vi "Day1-b.vi"(10 "Input":string="15931\n8782\n16940\n14614\n\n4829\n12415\n13259\n11441\n8199\n\n2540\n2500\n6341\n2235\n1858\n4157\n5053\n6611\n1050\n4401\n6187\n1078\n3297\n\n25264\n23014\n15952\n\n10156\n4544\n4930\n11786\n15822\n\n1264\n6399\n2031\n6892\n3115\n5151\n5093\n6724\n7001\n4011\n1458\n1945\n\n2106\n2016\n1528\n2524\n6089\n4466\n3154\n2686\n3289\n5831\n1520\n2122\n5744\n\n33066\n22616\n\n1993\n8485\n1037\n9730\n2076\n7492\n10000\n2971\n\n11027\n9137\n4599\n7461\n1531\n12939\n\n17530\n18837\n19466\n4845\n\n1467\n4870\n10176\n6657\n5608\n2096\n9977\n6478\n\n18828\n26577\n\n17901\n5059\n13789\n4993\n\n6676\n3415\n2464\n5937\n4275\n6629\n7566\n1943\n6313\n4572\n\n9121\n10713\n5071\n1669\n7736\n10522\n6231\n\n6400\n1771\n4568\n7681\n7486\n60...") -> (2 "Output":i32)   [LabVIEW 2017]
uses:
  OOP/Elf/Elf.lvclass
  OOP/ElfHeap/ElfHeap.lvclass
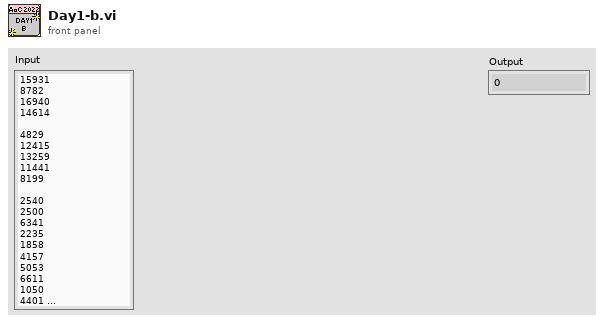
[diagram p1: front panel]
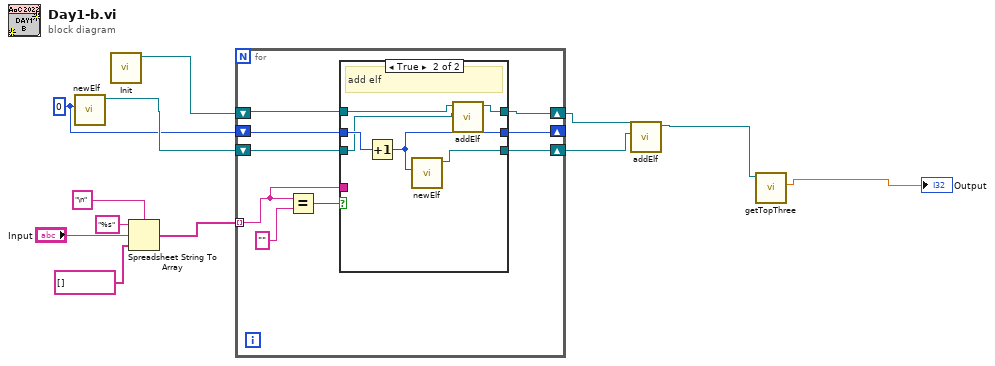
[diagram p0: block diagram]
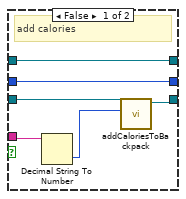
[diagram p2: hidden frame]
diagram:
  w6 = 0 ("Index")
  n1 = call "newElf.vi"("Index"=w6) -> ("Elf out"=w7:refnum<class "Elf.lvclass">)  [unwired: 9 in, 1 out]
  n2 = call "Init.vi"() -> ("ElfHeap out"=w5:refnum<class "ElfHeap.lvclass">)  [unwired: 10 in, 1 out]
  n3 = Spreadsheet String To Array(delimiter (Tab)="\n", format string="%s", spreadsheet string="Input", array type (2D Dbl)=string[] []) -> (array=w9:string[])
  n4 = for {
    tunnel: w9 -> [w13] mode=indexing
    shift-right: [w19] -> w4
    shift-left: w5 -> [w18]
    shift-right: [w16] -> _
    shift-left: w6 -> [w15]
    shift-right: [w14] -> w3
    shift-left: w7 -> [w17]
    n5 = Equal?(x=w13, y="" ("delimiter (Tab)")) -> (x = y?=w20:bool)
    n6 = case shown="True" w20 {
      tunnel: [w27 w28] -> w19
      tunnel: w18 -> [w27 w30]
      tunnel: w17 -> [w25 w29]
      tunnel: [w26 w32] -> w16
      tunnel: w15 -> [w26 w33]
      tunnel: [w24 w31] -> w14
      tunnel: w13 -> [w23 _]
      frame False {
        # "add calories"
        n7 = Decimal String To Number(string=w23) -> (number=w22:i32)  [unwired: 2 in, 1 out]
        n8 = call-dynamic "addCaloriesToBackpack.vi"("Calories"=w22, "Elf in"=w25) -> ("Elf out"=w24:refnum<class "Elf.lvclass">)  [unwired: 8 in, 1 out]
      }
      frame True {
        # "add elf"
        n9 = Increment(x=w33) -> (x+1=w32:i32)
        n10 = call "newElf.vi"("Index"=w32) -> ("Elf out"=w31:refnum<class "Elf.lvclass">)  [unwired: 9 in, 1 out]
        n11 = call-dynamic "addElf.vi"("Elf.lvclass"=w29, "ElfHeap in"=w30) -> ("ElfHeap out"=w28:refnum<class "ElfHeap.lvclass">)  [unwired: 8 in, 1 out]
      }
    }
  }
  n12 = call-dynamic "addElf.vi"("Elf.lvclass"=w3, "ElfHeap in"=w4) -> ("ElfHeap out"=w2:refnum<class "ElfHeap.lvclass">)  [unwired: 8 in, 1 out]
  n13 = call-dynamic "getTopThree.vi"("ElfHeap in"=w2) -> ("Sum Top Three Carried Calories"=→"Output":dbl)  [unwired: 9 in, 1 out]
